vi "Init UI.vi"(8 "error in (no error)":errorcluster, 11 "LF2R IDE in":refnum<class "Main Panel.lvclass">) -> (0 "error out":errorcluster, 3 "LF2R IDE out":refnum<class "Main Panel.lvclass">)   [LabVIEW 2018, in "Main Panel.lvlib" / "Main Panel.lvclass"]
uses:
  Main Panel.lvclass
  Main Panel.lvclass/Main Panel.ctl
  Framework/Framework/Framework.lvclass
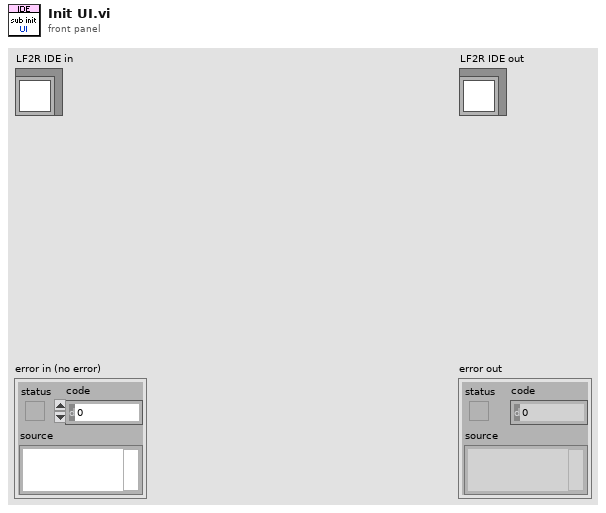
[diagram p1: front panel]
types:
  T1 = typedef "Framework.lvlib/Framework.lvclass/Const Lang Setting.ctl" = cluster{"Main Panel":T2, "Configuration Window":T15}
  T2 = typedef "Framework.lvlib/Framework.lvclass/Const Lang MainWnd.ctl" = cluster{"Title":T3, "Frame Basic":T5, "Frame Skill":T6, "bp":T7, "w":T8, "b":T9, "i":T10, "o":T11, "c":T12, "Other":T13, "Menu":T14}
  T3 = typedef "Framework.lvlib/Framework.lvclass/Const Lang MainWnd Frame Title.ctl" = cluster{"Frame Num":T4, "Name":T4}
  T4 = typedef "Framework.lvlib/Framework.lvclass/Const Lang Property.ctl" = cluster{"Name":string, "Tip":string, "Description":string}
  T5 = typedef "Framework.lvlib/Framework.lvclass/Const Lang MainWnd Frame Basic.ctl" = cluster{"pic":T4, "state":T4, "wait":T4, "next":T4, "dvx":T4, "dvy":T4, "dvz":T4, "centerx":T4, "centery":T4, "sound":T4}
  T6 = typedef "Framework.lvlib/Framework.lvclass/Const Lang MainWnd Frame Skill.ctl" = cluster{"mp":T4, "hit_a":T4, "hit_d":T4, "hit_j":T4, "hit_Fa":T4, "hit_Ua":T4, "hit_Da":T4, "hit_Fj":T4, "hit_Uj":T4, "hit_Dj":T4, "hit_ja":T4}
  T7 = typedef "Framework.lvlib/Framework.lvclass/Const Lang MainWnd Frame bp.ctl" = cluster{"x":T4, "y":T4}
  T8 = typedef "Framework.lvlib/Framework.lvclass/Const Lang MainWnd Frame w.ctl" = cluster{"kind":T4, "x":T4, "y":T4, "weaponact":T4, "cover":T4, "dvx":T4, "dvy":T4, "dvz":T4, "attacking":T4}
  T9 = typedef "Framework.lvlib/Framework.lvclass/Const Lang MainWnd Frame b.ctl" = cluster{"kind":T4, "x":T4, "y":T4, "w":T4, "h":T4, "index":T4}
  T10 = typedef "Framework.lvlib/Framework.lvclass/Const Lang MainWnd Frame i.ctl" = cluster{"kind":T4, "x":T4, "y":T4, "w":T4, "h":T4, "zwidth":T4, "dvx":T4, "dvy":T4, "dvz":T4, "fall":T4, "arest":T4, "vrest":T4, "bdefend":T4, "injury":T4, "effect":T4, "catchingact 1":T4, "catchingact 2":T4, "caughtact 1":T4, "caughtact 2":T4, "index":T4}
  T11 = typedef "Framework.lvlib/Framework.lvclass/Const Lang MainWnd Frame o.ctl" = cluster{"kind":T4, "x":T4, "y":T4, "action":T4, "dvx":T4, "dvy":T4, "dvz":T4, "oid":T4, "facing":T4}
  T12 = typedef "Framework.lvlib/Framework.lvclass/Const Lang MainWnd Frame c.ctl" = cluster{"kind":T4, "x":T4, "y":T4, "injury":T4, "cover":T4, "vaction":T4, "aaction":T4, "taction":T4, "hurtable":T4, "decrease":T4, "fronthurtact":T4, "backhurtact":T4, "throwvx":T4, "throwvy":T4, "throwvz":T4, "throwinjury":T4, "dircontrol":T4}
  T13 = typedef "Framework.lvlib/Framework.lvclass/Const Lang MainWnd Other.ctl" = cluster{"File Path":T4, "GoTo":T4, "Apply Change":T4, "To Next Frame":T4, "Sound Play":T4}
  T14 = typedef "Framework.lvlib/Framework.lvclass/Const Lang MainWnd Menu.ctl" = cluster{"File":T4, "Open File":T4, "Save File":T4, "Exit":T4, "Settings":T4, "Preferences":T4, "Help":T4, "Show Context Help":T4}
  T15 = typedef "Framework.lvlib/Framework.lvclass/Const Lang CfgWnd.ctl" = cluster{"Tab":T16, "Main":T17, "Path":T18, "Image":T19}
  T16 = typedef "Framework.lvlib/Framework.lvclass/Const Lang CfgWnd Tab.ctl" = cluster{"Main Page":T4, "Image Page":T4}
  T17 = typedef "Framework.lvlib/Framework.lvclass/Const Lang CfgWnd Main.ctl" = cluster{"Language":T4, "Save":T4, "Cancel":T4}
  T18 = typedef "Framework.lvlib/Framework.lvclass/Const Lang CfgWnd Path.ctl" = cluster{"Reset":T4, "Path Data":T4, "Path Png":T4, "Path Mp3":T4}
  T19 = typedef "Framework.lvlib/Framework.lvclass/Const Lang CfgWnd Image.ctl" = cluster{"Center Point":cluster{"Name":T4, "Size":T4, "Color":T4, "Enable":T4}, "bp Point":cluster{"Name":T4, "Size":T4, "Color":T4, "Enable":T4}, "w Point":cluster{"Name":T4, "Size":T4, "Color":T4, "Enable":T4}, "b Box":cluster{"Name":T4, "Fill Color":T4, "Border Color":T4, "Enable":T4}, "i Box":cluster{"Name":T4, "Fill Color":T4, "Border Color":T4, "Enable":T4}, "o Point":cluster{"Name":T4, "Size":T4, "Color":T4, "Enable":T4}, "c Point":cluster{"Name":T4, "Size":T4, "Color":T4, "Enable":T4}}
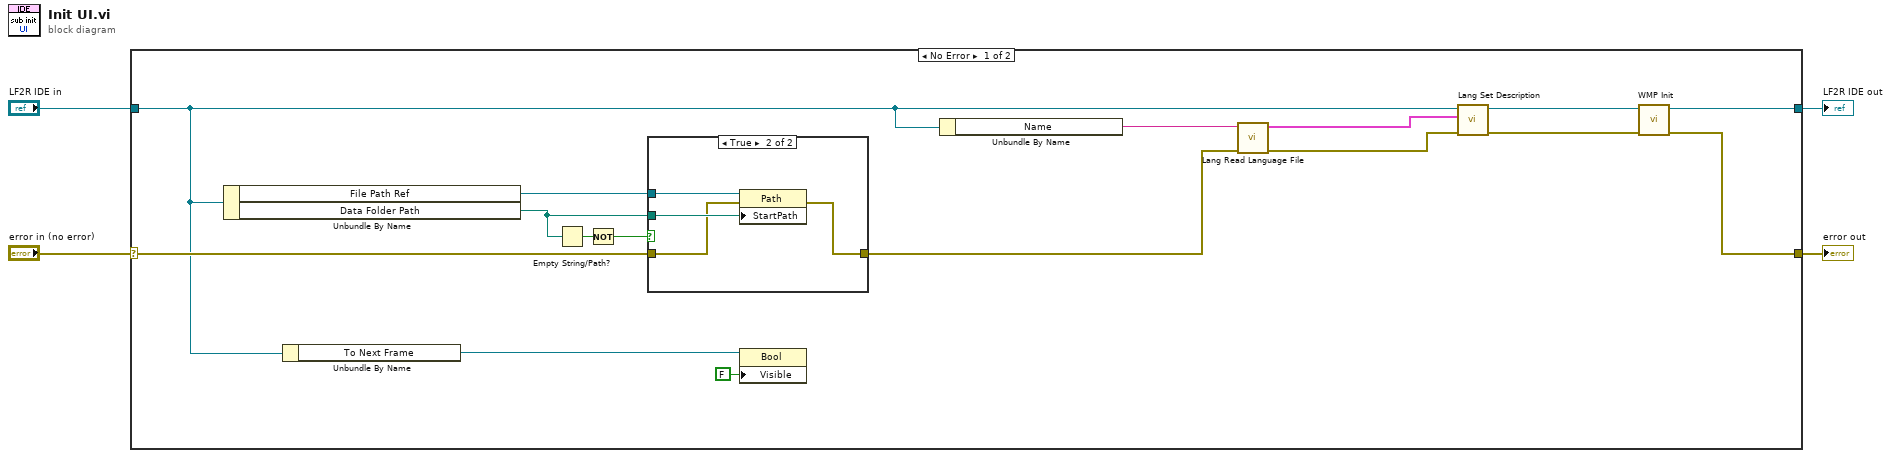
[diagram p0: block diagram]
diagram:
  n1 = case shown="No Error" "error in (no error)" {
    selector: "error in (no error)" -> [w19 w27]
    tunnel: [w9 w27] -> w3
    tunnel: [w11 w26] -> w1
    tunnel: "LF2R IDE in" -> [w7 w26]
    frame No Error {
      n2 = Unbundle By Name(w7) -> ("File Path Ref"=w20:refnum<vi>, "Data Folder Path"=w18:path)
      n3 = Unbundle By Name(w7) -> ("To Next Frame"=w6:refnum<vi>)
      n4 = Empty String/Path?(string/path=w18) -> (empty?=w17:bool)
      n5 = Not(x=w17) -> (.not. x?=w16:bool)
      n6 = case shown="True" w16 {
        tunnel: w20 -> [_ w25]
        tunnel: [w21 w24] -> w8
        tunnel: w18 -> [_ w23]
        tunnel: w19 -> [w21 w22]
        frame False {
        }
        frame True {
          n7 = property class="Path"(reference=w25, error in=w22, "StartPath"=w23) -> (error out=w24:errorcluster)  [unwired: 1 out]
        }
      }
      n8 = property class="Bool"(reference=w6, "Visible"=FALSE) -> ()  [unwired: 1 in, 2 out]
      n9 = Unbundle By Name(w7) -> ("Name"=w14:string)
      n10 = call "Lang Read Language File.vi"("error in (no error)"=w8, "Language Name"=w14) -> ("error out"=w15:errorcluster, "UI Descriptions"=w13:T1)  [unwired: 7 in, 1 out]
      n11 = call "Lang Set Description.vi"("error in (no error)"=w15, "UI Descriptions"=w13, "LF2R IDE in"=w7) -> ("error out"=w10:errorcluster, "LF2R IDE out"=w12:refnum<class "Main Panel.lvclass">)  [unwired: 7 in]
      n12 = call "WMP Init.vi"("error in (no error)"=w10, "Main Panel in"=w12) -> ("error out"=w9:errorcluster, "Main Panel out"=w11:refnum<class "Main Panel.lvclass">)  [unwired: 8 in]
    }
    frame Error {
    }
  }
  "error out" <- w3
  "LF2R IDE out" <- w1
